vi "lock - unlock user license.vi"(8 "error in (no error)":errorcluster, 9 "User Record":T1={"ixUser"=0, "sxUsername"="", "sLastName"="", "sFirstName"="", "sEmail"="", "sPassword"="", "tLoginTime"=timestamp(0 s since 1904-01-01), "sLoginComputer"="", "fAdministrator"=FALSE, "fRunSequences"=TRUE, "fModifySequences"=FALSE, "fRunScenarios"=FALSE, "fModifyScenarios"=FALSE, "fModifyTemplates"=FALSE, "fModifyUsers"=FALSE, "fModifyStations"=FALSE, "fModifyFields"=FALSE}, 10 "Action":enum16{"Lock", "Unlock"}(ring), 11 "Connection Refnum":T2) -> (0 "error out":errorcluster, 3 "Connection Refnum":T2)   [LabVIEW 2011]
uses:
  SI.LIB/ODBC/SQL Controls/Connection Refnum.ctl
  server/database/Users/User Record.ctl
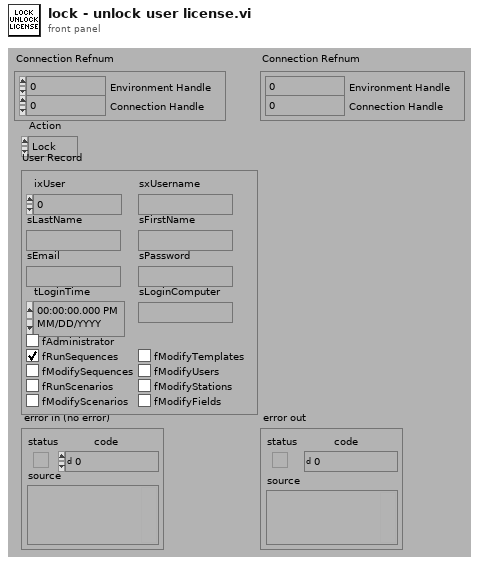
[diagram p1: front panel]
types:
  T1 = typedef "User Record.ctl" = cluster{"ixUser":i32, "sxUsername":string, "sLastName":string, "sFirstName":string, "sEmail":string, "sPassword":string, "tLoginTime":timestamp, "sLoginComputer":string, "fAdministrator":bool, "fRunSequences":bool, "fModifySequences":bool, "fRunScenarios":bool, "fModifyScenarios":bool, "fModifyTemplates":bool, "fModifyUsers":bool, "fModifyStations":bool, "fModifyFields":bool}
  T2 = typedef "Connection Refnum.ctl" = cluster{"Environment Handle":i32, "Connection Handle":i32}
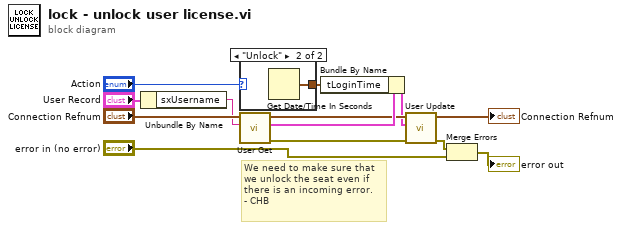
[diagram p0: block diagram]
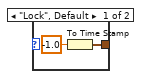
[diagram p2: hidden frame]
diagram:
  # "We need to make sure that\nwe unlock the seat even if\nthere is an incoming error.\n- CHB"
  n1 = Unbundle By Name("User Record") -> ("sxUsername"=w1:string)
  n2 = case shown="\"Unlock\"" "Action" {
    tunnel: [w14 w16] -> w10
    frame "Lock", Default {
      n3 = To Time Stamp(1:-1.0 ("number")) -> (0:w14:timestamp)
    }
    frame "Unlock" {
      n4 = Get Date/Time In Seconds() -> (seconds since 1Jan1904=w16:timestamp)
    }
  }
  n5 = call "User Get.vi"("sxUsername (\"\")"=w1, "Connection Refnum"="Connection Refnum") -> ("error out"=w7:errorcluster, "User"=w12:T1, "Connection Refnum"=w9:T2)  [unwired: 1 in, 6 out]
  n6 = Bundle By Name(cluster=w12, "tLoginTime"=w10) -> (w6:T1)
  n7 = call "User Update.vi"("error in (no error)"=w7, "User Record"=w6, "Connection Refnum"=w9) -> ("error out"=w5:errorcluster, "dup Connection Refnum"=→"Connection Refnum":T2)  [unwired: 7 out]
  n8 = Merge Errors(w5, "error in (no error)") -> (→"error out":errorcluster)
